vi "DEVICE_UNIT_SELECTOR - Type.vi"(8 "error in (no error)":errorcluster, 11 "DEVICE_UNIT_SELECTOR":T1) -> (0 "error out":errorcluster, 3 "DEVICE_UNIT_SELECTOR":i32)   [LabVIEW 2015]
doc: "<b>Camera LED state options.</b>\nHEARTBEAT : Blink if link is ok (led 1), heartbeat mode (led 2).\nTRIGGER_ACTIVE : Blink led if trigger detected.\nEXT_EVENT_ACTIVE : Blink led if external signal detected.\nACQUISITION : Blink led during data streaming.\nEXPOSURE_ACTIVE : Blink led during sensor integration time.\nFRAME_ACTIVE : Blink if device busy/not busy.\nLINK : Blink led if link is ok.\nOFF : Set led to zero.\nON : Set led to one."
uses:
  DEVICE_UNIT_SELECTOR.ctl
  C:/GIT/Cameras3.x/Integrations/Labview/xiLib/xiLIB_64bit/xiLIB/xiCamLib/API/x64/xiApi.NETX64.dll
  API/x64/xiApi.NETX64.dll
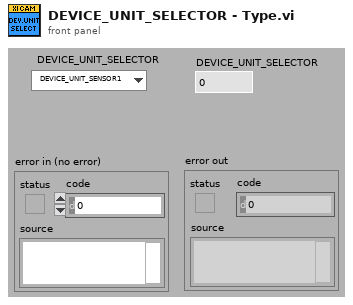
[diagram p1: front panel]
types:
  T1 = typedef "DEVICE_UNIT_SELECTOR.ctl" = enum16{"DEVICE_UNIT_SENSOR1", "DEVICE_UNIT_FPGA1", "DEVICE_UNIT_SAL", "DEVICE_UNIT_DAL", "DEVICE_UNIT_SCM", "DEVICE_UNIT_FGENTL", "DEVICE_UNIT_MCU1", "DEVICE_UNIT_MCU2", "DEVICE_UNIT_CHF"}
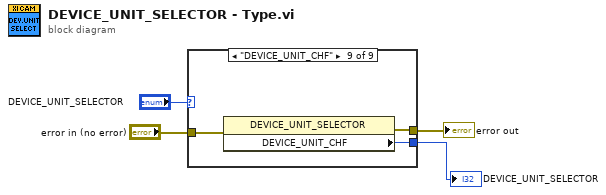
[diagram p0: block diagram]
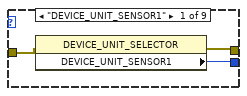
[diagram p2: hidden frame]
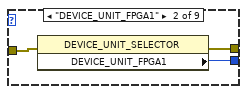
[diagram p3: hidden frame]
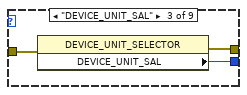
[diagram p4: hidden frame]
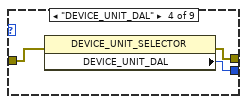
[diagram p5: hidden frame]
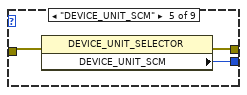
[diagram p6: hidden frame]
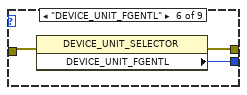
[diagram p7: hidden frame]
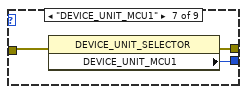
[diagram p8: hidden frame]
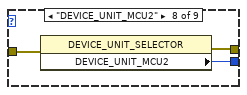
[diagram p9: hidden frame]
diagram:
  n1 = case shown="\"DEVICE_UNIT_CHF\"" "DEVICE_UNIT_SELECTOR" {
    tunnel: "error in (no error)" -> [w7 w10 w11 w16 w19 w22 w23 w26 w31]
    tunnel: [w6 w9 w12 w15 w18 w21 w24 w27 w30] -> w2
    tunnel: [w5 w8 w13 w14 w17 w20 w25 w28 w29] -> w1
    frame "DEVICE_UNIT_SENSOR1" {
      n2 = property class="DEVICE_UNIT_SELECTOR"(error in=w7) -> (error out=w6:errorcluster, "DEVICE_UNIT_SENSOR1"=w5:i32)  [unwired: 1 in, 1 out]
    }
    frame "DEVICE_UNIT_FPGA1" {
      n3 = property class="DEVICE_UNIT_SELECTOR"(error in=w10) -> (error out=w9:errorcluster, "DEVICE_UNIT_FPGA1"=w8:i32)  [unwired: 1 in, 1 out]
    }
    frame "DEVICE_UNIT_SAL" {
      n4 = property class="DEVICE_UNIT_SELECTOR"(error in=w11) -> (error out=w12:errorcluster, "DEVICE_UNIT_SAL"=w13:i32)  [unwired: 1 in, 1 out]
    }
    frame "DEVICE_UNIT_DAL" {
      n5 = property class="DEVICE_UNIT_SELECTOR"(error in=w16) -> (error out=w15:errorcluster, "DEVICE_UNIT_DAL"=w14:i32)  [unwired: 1 in, 1 out]
    }
    frame "DEVICE_UNIT_SCM" {
      n6 = property class="DEVICE_UNIT_SELECTOR"(error in=w19) -> (error out=w18:errorcluster, "DEVICE_UNIT_SCM"=w17:i32)  [unwired: 1 in, 1 out]
    }
    frame "DEVICE_UNIT_FGENTL" {
      n7 = property class="DEVICE_UNIT_SELECTOR"(error in=w22) -> (error out=w21:errorcluster, "DEVICE_UNIT_FGENTL"=w20:i32)  [unwired: 1 in, 1 out]
    }
    frame "DEVICE_UNIT_MCU1" {
      n8 = property class="DEVICE_UNIT_SELECTOR"(error in=w23) -> (error out=w24:errorcluster, "DEVICE_UNIT_MCU1"=w25:i32)  [unwired: 1 in, 1 out]
    }
    frame "DEVICE_UNIT_MCU2" {
      n9 = property class="DEVICE_UNIT_SELECTOR"(error in=w26) -> (error out=w27:errorcluster, "DEVICE_UNIT_MCU2"=w28:i32)  [unwired: 1 in, 1 out]
    }
    frame "DEVICE_UNIT_CHF" {
      n10 = property class="DEVICE_UNIT_SELECTOR"(error in=w31) -> (error out=w30:errorcluster, "DEVICE_UNIT_CHF"=w29:i32)  [unwired: 1 in, 1 out]
    }
  }
  "error out" <- w2
  "DEVICE_UNIT_SELECTOR" <- w1
